vi "InitFromXML.vi"(8 "error in (no error)":errorcluster, 10 "XML":string, 11 "GettingStartedWindow.lvlib:RunVI.lvclass":refnum<class "RunVI.lvclass">) -> (0 "error out":errorcluster, 3 "GettingStartedWindow.lvlib:RunVI.lvclass out":refnum<class "RunVI.lvclass">)   [LabVIEW 2009, in "NavScreen.lvlib" / "RunVI.lvclass"]
uses:
  RunVI.lvclass
  ClickableText/ClickableText.lvclass
  RunVI.lvclass/RunVI.ctl
  NavScreen.lvlib
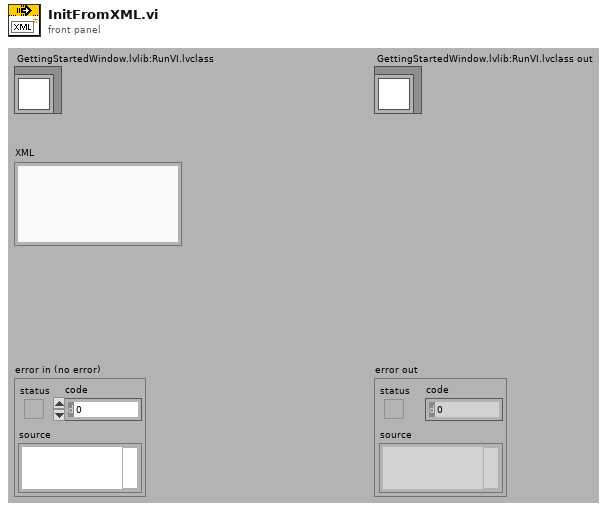
[diagram p1: front panel]
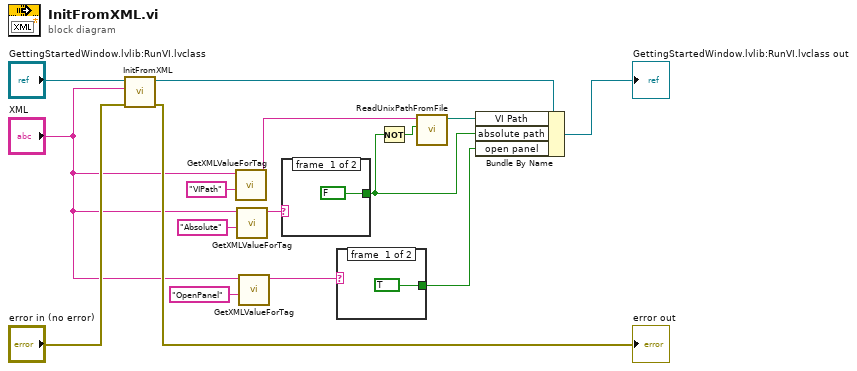
[diagram p0: block diagram]
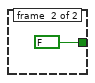
[diagram p2: hidden frame]
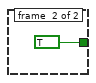
[diagram p3: hidden frame]
diagram:
  n1 = call-parent "InitFromXML.vi"("error in (no error)"="error in (no error)", "XML"="XML", "ClickableText in"="GettingStartedWindow.lvlib:RunVI.lvclass") -> ("error out"=→"error out":errorcluster, "ClickableText out"=w13:refnum<class "RunVI.lvclass">)  [unwired: 7 in]
  n2 = call "GetXMLValueForTag.vi"("tag"="VIPath", "XML"="XML") -> ("value"=w10:string)  [unwired: 8 in, 1 out]
  n3 = call "GetXMLValueForTag.vi"("tag"="Absolute", "XML"="XML") -> ("value"=w7:string)  [unwired: 8 in, 1 out]
  n4 = call "GetXMLValueForTag.vi"("tag"="OpenPanel", "XML"="XML") -> ("value"=w4:string)  [unwired: 8 in, 1 out]
  n5 = case shown="Default" w7 {
    tunnel: [FALSE TRUE] -> w2
    frame #0 {
    }
    frame #1 {
    }
  }
  n6 = case shown="Default" w4 {
    tunnel: [TRUE FALSE] -> w3
    frame #0 {
    }
    frame #1 {
    }
  }
  n7 = Not(x=w2) -> (.not. x?=w1:bool)
  n8 = call "ReadUnixPathFromFile.vi"("relative"=w1, "path"=w10) -> ("path"=w9:path)  [unwired: 9 in]
  n9 = Bundle By Name(cluster=w13, "VI Path"=w9, "absolute path"=w2, "open panel"=w3) -> (→"GettingStartedWindow.lvlib:RunVI.lvclass out":refnum<class "RunVI.lvclass">)
